vi "SpreadsheetdataanalysisJ&J.vi"() -> (1 "Decay Plot":cluster{"all rows":dbl[], "all rows":dbl[]}(graph))   [LabVIEW 2015]
uses:
  <vilib>/Utility/file.llb/Read Delimited Spreadsheet (DBL).vi
  <vilib>/Analysis/NI_AALBase.lvlib
panel:
  out "Poisson Histogram":T1(graph)
  out "Decay Plot w/Exponential Fit":cluster{"all rows":dbl[], "all rows":dbl[]}[](graph)
  out "Acquisition Time (s)":cluster{"Column 0":dbl[], "Column 1":dbl[]}
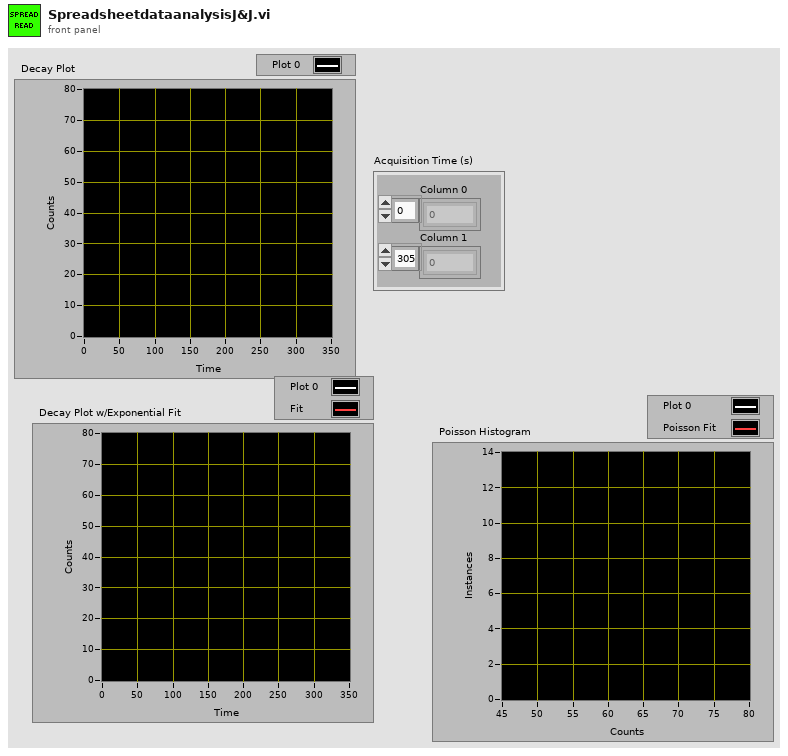
[diagram p1: front panel]
types:
  T1 = cluster{"X Values":dbl[], "Histogram: h(x)":i32[]}[]
  T2 = cluster{"X Values":dbl[], "Histogram: h(x)":i32[]}
  T3 = cluster{"Array":dbl[], "Histogram: h(x)":i32[]}[]
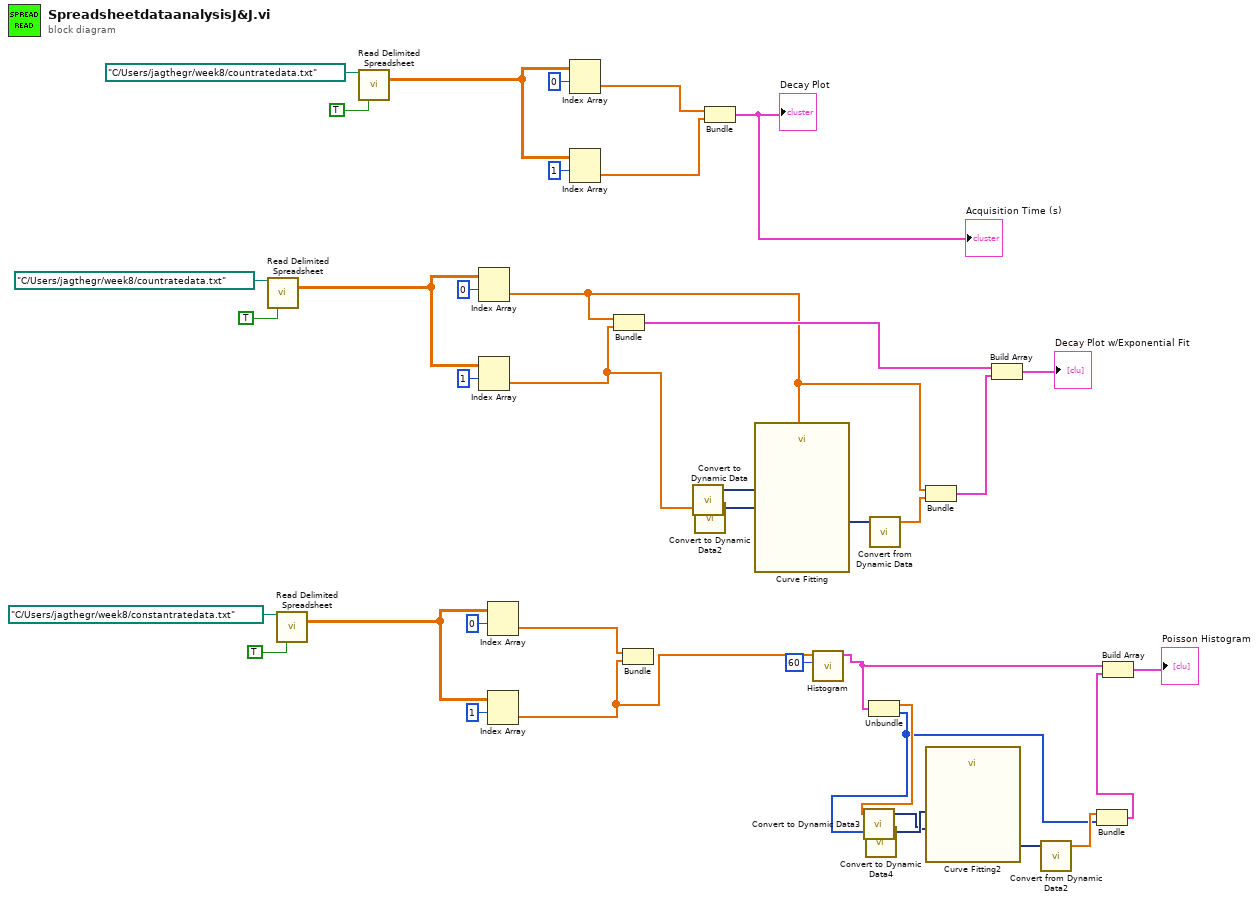
[diagram p0: block diagram]
diagram:
  n1 = call-poly <vilib>:"Read Delimited Spreadsheet.vi"("file path (dialog if empty)"=path "C:/Users/jagthegr/week8/countratedata.txt", "transpose? (F)"=TRUE) -> ("all rows"=w29:dbl[][])  [unwired: 8 in, 5 out]
  n2 = call-poly <vilib>:"Read Delimited Spreadsheet.vi"("file path (dialog if empty)"=path "C:/Users/jagthegr/week8/constantratedata.txt", "transpose? (F)"=TRUE) -> ("all rows"=w24:dbl[][])  [unwired: 8 in, 5 out]
  n3 = call-poly <vilib>:"Read Delimited Spreadsheet.vi"("file path (dialog if empty)"=path "C:/Users/jagthegr/week8/countratedata.txt", "transpose? (F)"=TRUE) -> ("all rows"=w37:dbl[][])  [unwired: 8 in, 5 out]
  n4 = Index Array(array=w29, index (row)=0 ("index")) -> (element=w14:dbl[])  [unwired: 1 in]
  n5 = Index Array(array=w29, index (row)=1 ("index")) -> (element=w18:dbl[])  [unwired: 1 in]
  n6 = Index Array(array=w24, index (row)=0 ("index")) -> (element=w2:dbl[])  [unwired: 1 in]
  n7 = Index Array(array=w24, index (row)=1 ("index")) -> (element=w12:dbl[])  [unwired: 1 in]
  n8 = Index Array(array=w37, index (row)=0 ("index")) -> (element=w36:dbl[])  [unwired: 1 in]
  n9 = Index Array(array=w37, index (row)=1 ("index")) -> (element=w35:dbl[])  [unwired: 1 in]
  n10 = Bundle("all rows"=w14, "all rows"=w18) -> (w17:cluster{"all rows":dbl[], "all rows":dbl[]})  [unwired: 1 in]
  n11 = Bundle("all rows"=w2, "all rows"=w12) -> ()  [unwired: 1 in, 1 out]
  n12 = call "Convert to Dynamic Data"("Array"=w14) -> ("Dynamic Data Type"=w21:dynamicdata)  [unwired: 3 in]
  n13 = call "Convert to Dynamic Data2"("Array"=w18) -> ("Dynamic Data Type"=w20:dynamicdata)  [unwired: 3 in]
  n14 = Bundle("all rows"=w36, "all rows"=w35) -> (→"Decay Plot" →"Acquisition Time (s)":cluster{"all rows":dbl[], "all rows":dbl[]})  [unwired: 1 in]
  n15 = call "Curve Fitting"("Locations"=w21, "Signals"=w20) -> ("best fit"=w19:dynamicdata)  [unwired: 6 in, 3 out]
  n16 = call <vilib>:"Histogram.vi"("intervals"=60, "X"=w12) -> ("Histogram Graph"=w5:T2)  [unwired: 6 in, 3 out]
  n17 = Unbundle(w5) -> ("X Values"=w10:dbl[], "Histogram: h(x)"=w3:i32[])
  n18 = call "Convert to Dynamic Data3"("Array"=w10) -> ("Dynamic Data Type"=w8:dynamicdata)  [unwired: 3 in]
  n19 = call "Convert to Dynamic Data4"("Array"=w3) -> ("Dynamic Data Type"=w9:dynamicdata)  [unwired: 3 in]
  n20 = call "Convert from Dynamic Data"("Dynamic Data Type"=w19) -> ("Array"=w15:dbl[])  [unwired: 3 in]
  n21 = Bundle("all rows"=w14, "Array"=w15) -> (w13:cluster{"all rows":dbl[], "Array":dbl[]})  [unwired: 1 in]
  n22 = call "Curve Fitting2"("Locations"=w9, "Signals"=w8) -> ("best fit"=w11:dynamicdata)  [unwired: 6 in, 3 out]
  n23 = Build Array(w17, w13) -> (→"Decay Plot w/Exponential Fit":cluster{"all rows":dbl[], "Array":dbl[]}[])
  n24 = call "Convert from Dynamic Data2"("Dynamic Data Type"=w11) -> ("Array"=w4:dbl[])  [unwired: 3 in]
  n25 = Bundle("Array"=w4, "Histogram: h(x)"=w3) -> (w6:cluster{"Array":dbl[], "Histogram: h(x)":i32[]})  [unwired: 1 in]
  n26 = Build Array(w5, w6) -> (→"Poisson Histogram":T3)
